vi "Get Primary Key.vi"(8 "error in (no error)":errorcluster, 11 "Basic Column Configuration in":refnum<class "Basic Column Configuration.lvclass">) -> (0 "error out":errorcluster, 2 "Is a PK?":bool, 3 "Basic Column Configuration out":refnum<class "Basic Column Configuration.lvclass">)   [LabVIEW 2020, in "Basic Columns.lvlib" / "Basic Column Configuration.lvclass"]
uses:
  Basic Column Configuration.lvclass
  Basic Column Configuration.lvclass/Basic Column Configuration.ctl
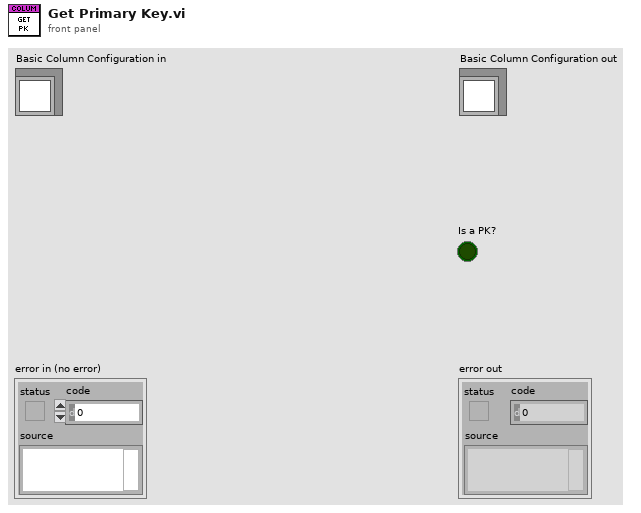
[diagram p1: front panel]
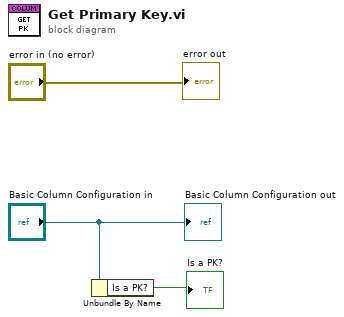
[diagram p0: block diagram]
diagram:
  n1 = Unbundle By Name("Basic Column Configuration in") -> ("Is a PK?"=→"Is a PK?":bool)
  "error out" <- "error in (no error)"
  "Basic Column Configuration out" <- "Basic Column Configuration in"
